vi "Main.vi"() -> ()   [LabVIEW 2021, in "Example Plugin.lvlib"]
doc: "This template is for the Queued Message Handler design pattern.\n\nThe Event Handling Loop generates messages based on user interface actions.\n\nThe Message Handling Loop processes messages generated by the Event Handling Loop, or by other messages. The messages are string values, so new messages can be added easily to the Message Cases case structure in the Message Handling Loop. Each message cluster can also provide an optional value for Message Data, which is a variant that can be converted to whatever message-specific data is required."
uses:
  Example Plugin.lvlib
  <vilib>/Plug-In SDKs/InstrumentStudio SDK/InstrumentStudioPluginSDK.lvlibp/Plugin Events Enum.ctl
  controls/Configuration.ctl
  377644f2-3ba0-40c2-9637-345728516e3e.vi
  dd0e9e37-20d8-45cf-b11e-f419cd56f172.vi
  377644f2-3ba0-40c2-9637-345728516e3e.vi/6651a77e-856e-4bcd-af5a-c0c13b264cc1.vi
  dd0e9e37-20d8-45cf-b11e-f419cd56f172.vi/331b549c-fcf8-43d9-8a1e-5b3c0091a99c.vi
  subVIs/Message Queue/Enqueue Message (Single).vi
  <vilib>/JDP Science/JSONtext/JSON text to Variant.vi
  <vilib>/Utility/error.llb/Error Cluster From Error Code.vi
  <vilib>/Plug-In SDKs/InstrumentStudio SDK/InstrumentStudioPluginSDK.lvlibp/Read Run Time Configuration.vi
  <vilib>/Plug-In SDKs/InstrumentStudio SDK/InstrumentStudioPluginSDK.lvlibp/Write Run Time Configuration.vi
  <vilib>/JDP Science/JSONtext/Variant to JSON Text.vi
  <vilib>/JDP Science/JSONtext/LVClass Serializer/JSONtext LVClass Serializer.lvclass
  <vilib>/ErrorRing/Error Ring.xnode
  <vilib>/Plug-In SDKs/InstrumentStudio SDK/InstrumentStudioPluginSDK.lvlibp/Plugin Session.lvclass
  <vilib>/Plug-In SDKs/InstrumentStudio SDK/InstrumentStudioPluginSDK.lvlibp
panel:
  in  "Tab Control 2":T1(tab)
  out "Project Path":path
  in  "Run Write":string
  in  "Write Run Time Config":bool
  in  "Edit Write":string
  in  "Write Edit Time Config":bool
  out "Run Read":string
  in  "Read Run Time Config":bool
  out "Edit Read":string
  in  "Read Edit Time Config":bool
  in  "Read Project Path":bool
  in  "Running":bool
  out "Event Record":i32(listbox)
  in  "Session Id":u64
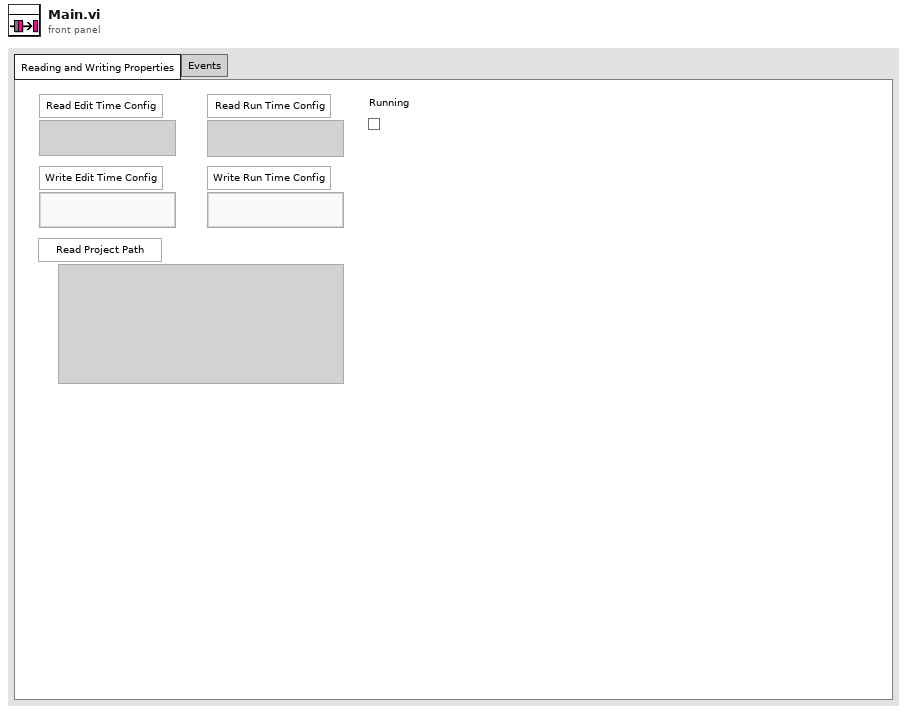
[diagram p1: front panel]
types:
  T1 = enum32{"Reading and Writing Properties", "Events"}
  T2 = typedef "Example Plugin.lvlib/Configuration.ctl" = cluster{"Edit Time Config":string, "Run Time Config":string, "Project Path":path}
  T3 = typedef "InstrumentStudioPluginSDK.lvlibp/Plugin Events Enum.ctl" = enum16{"Shutdown", "Project Saved", "Stop All Outputs"}
  T4 = typedef "InstrumentStudioPluginSDK.lvlibp/Event Registration Refnum.ctl" = refnum<event-registration>
  T5 = typedef "Example Plugin.lvlib/All Message Queues.ctl" = cluster{"UI":refnum<queue>}
  T6 = cluster{"Event Refnum":T4, "Event Registration Refnum":refnum<event-registration>}
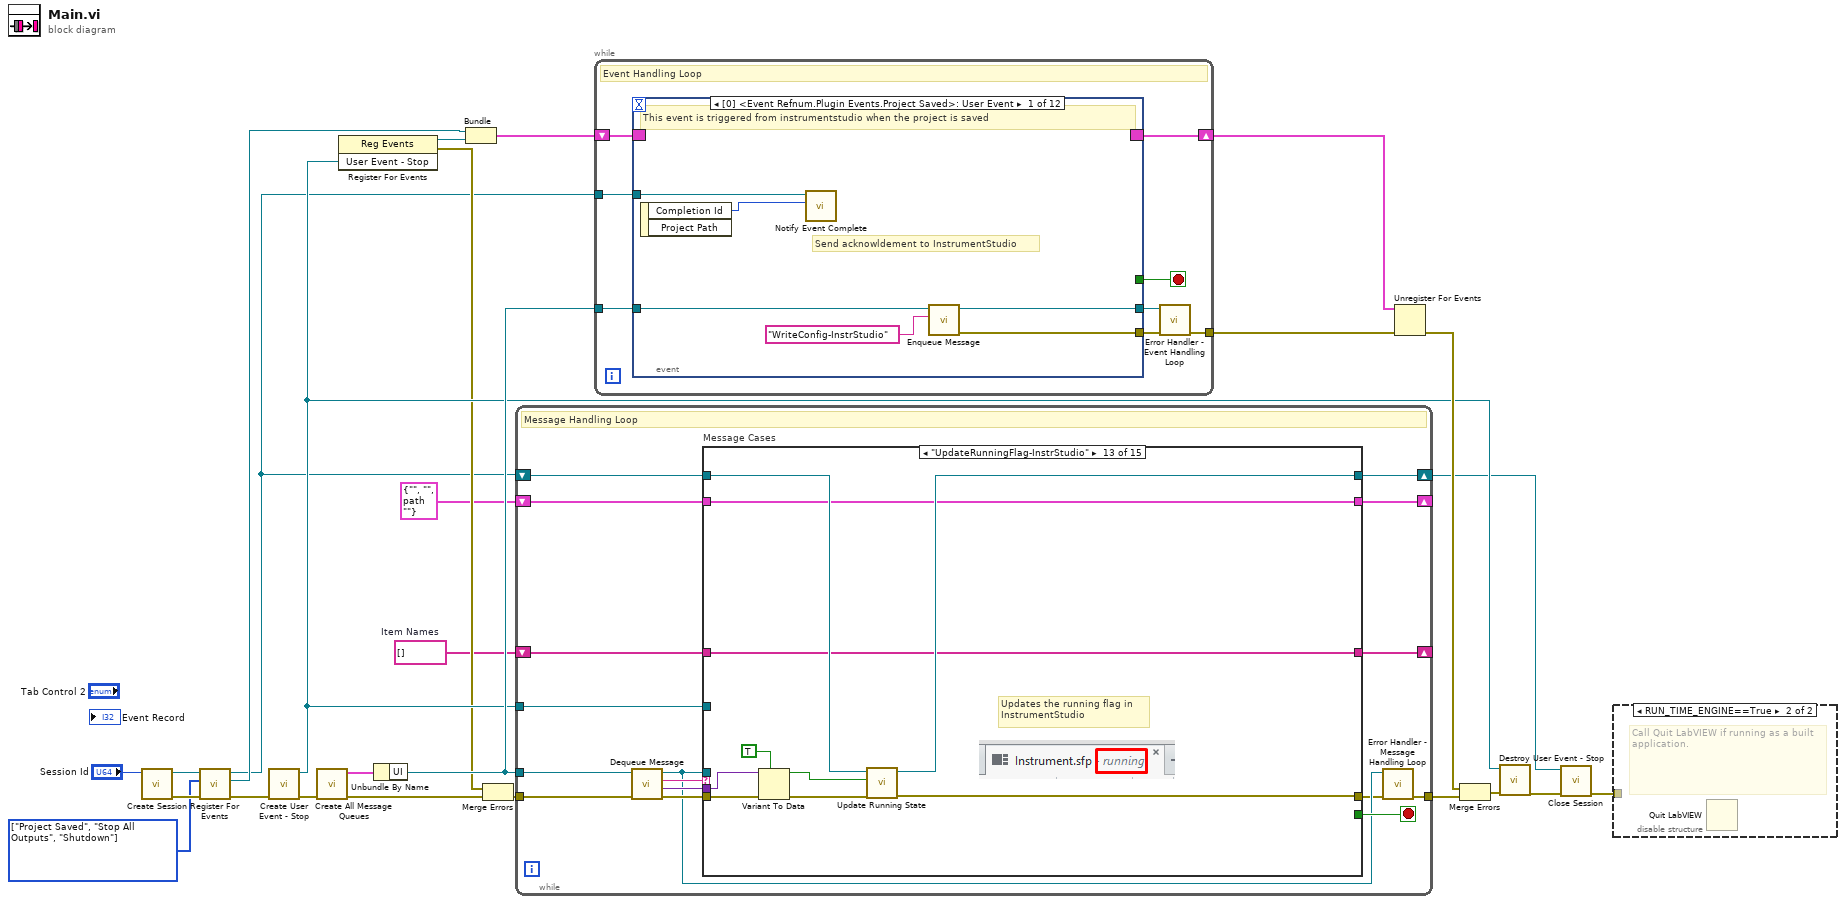
[diagram p0: block diagram]
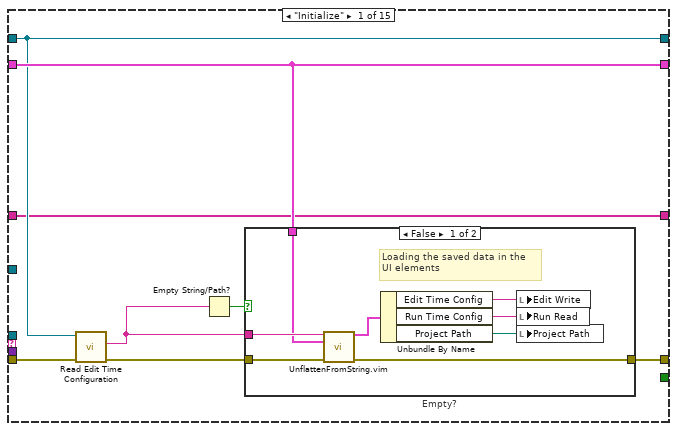
[diagram p3: hidden frame]
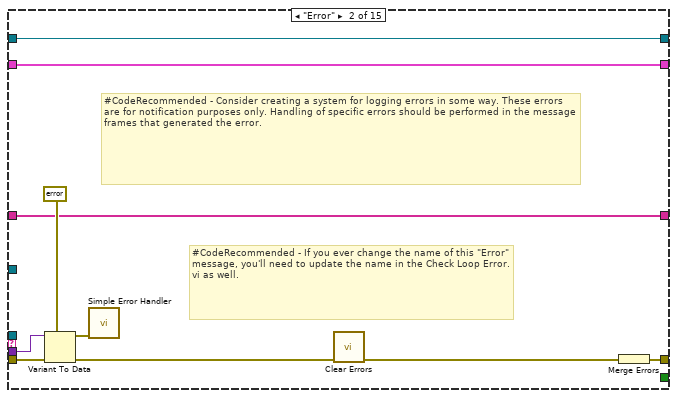
[diagram p5: hidden frame]
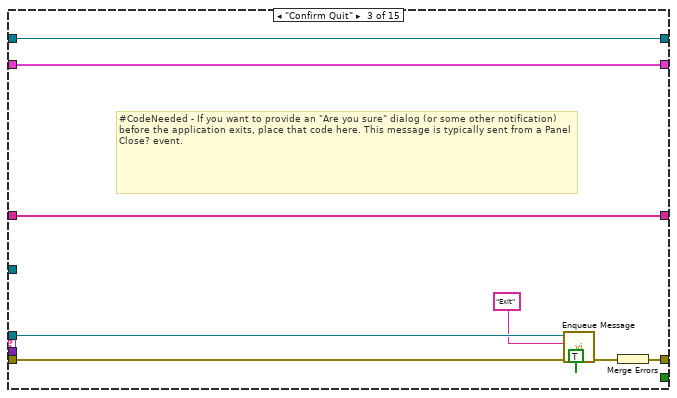
[diagram p6: hidden frame]
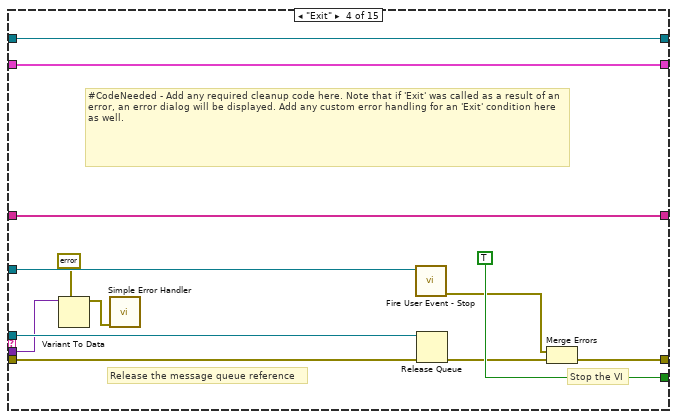
[diagram p7: hidden frame]
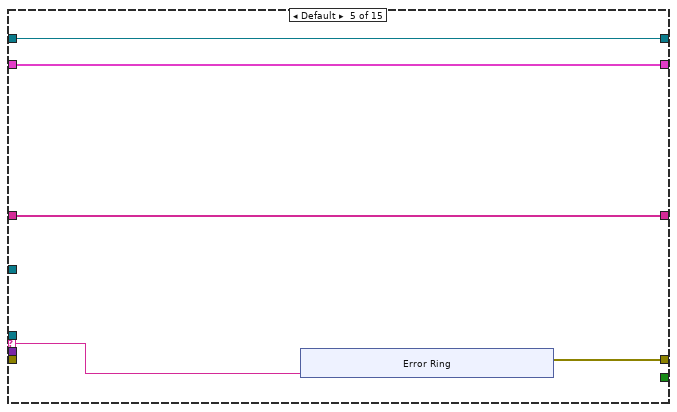
[diagram p8: hidden frame]
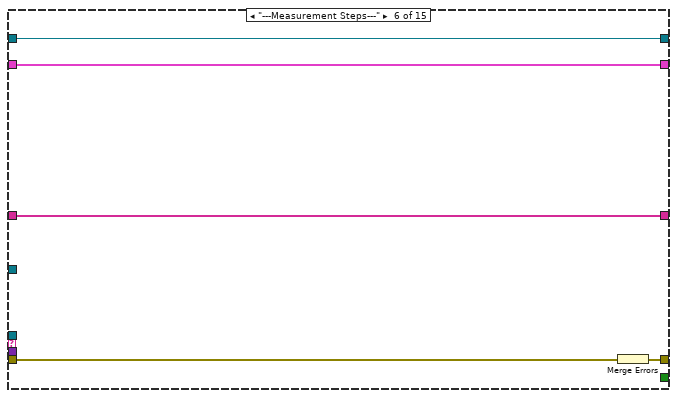
[diagram p9: hidden frame]
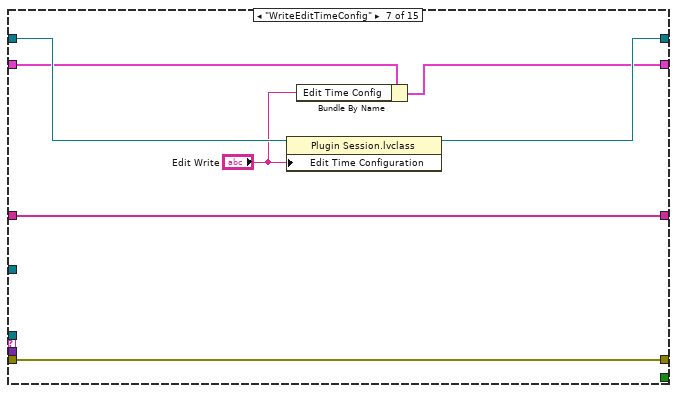
[diagram p10: hidden frame]
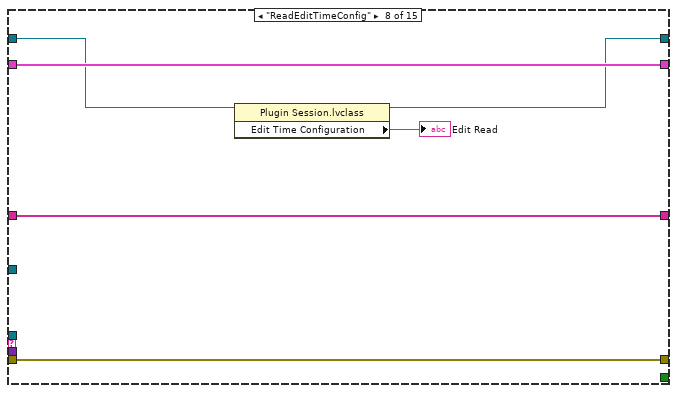
[diagram p11: hidden frame]
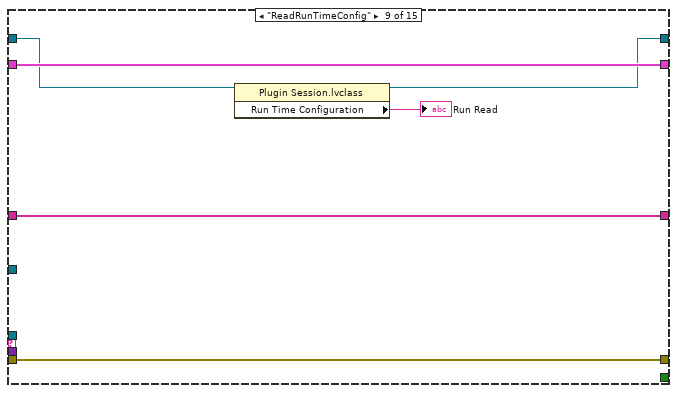
[diagram p12: hidden frame]
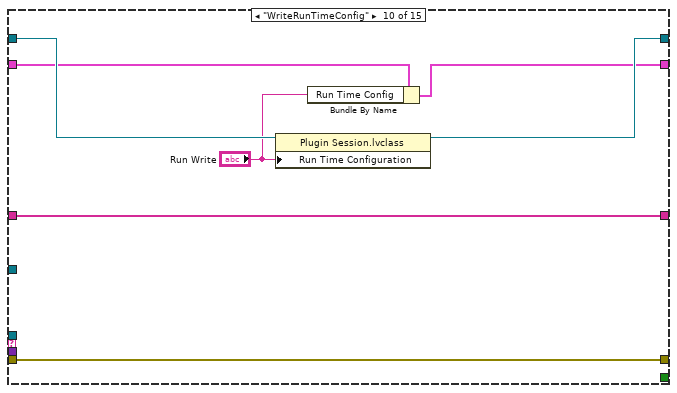
[diagram p13: hidden frame]
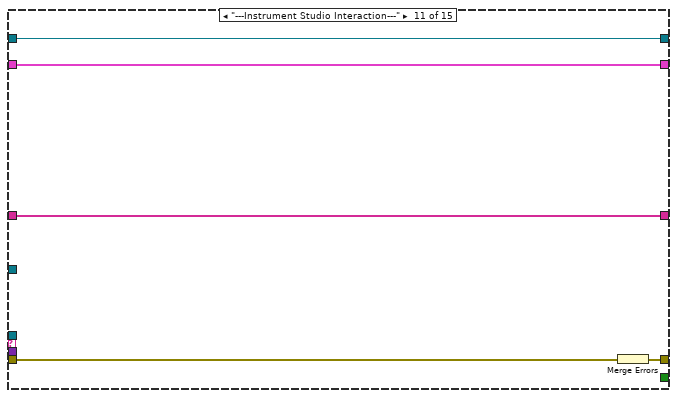
[diagram p14: hidden frame]
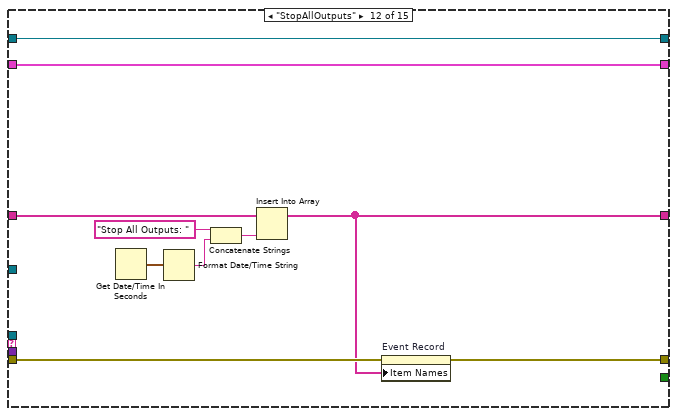
[diagram p15: hidden frame]
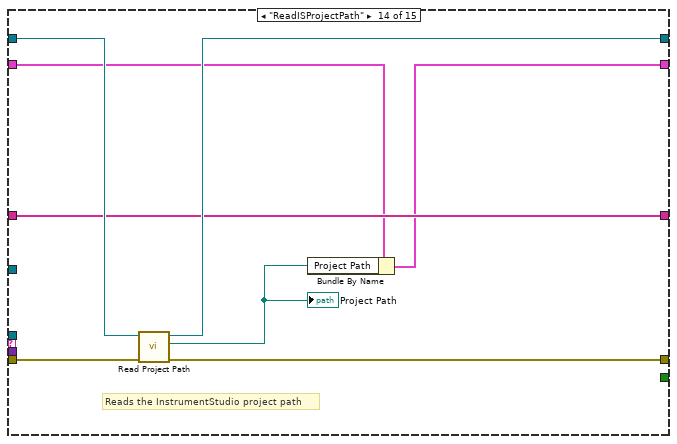
[diagram p16: hidden frame]
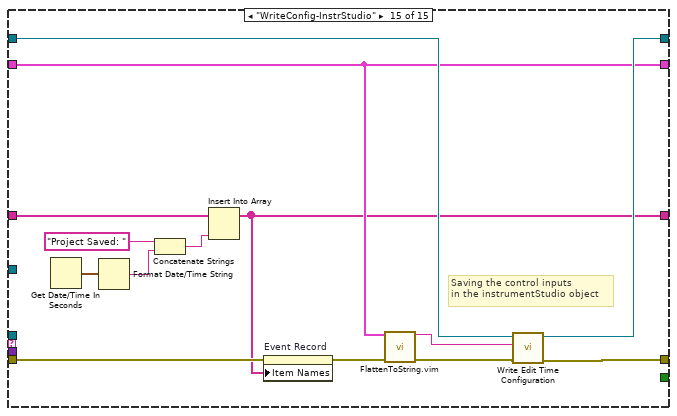
[diagram p17: hidden frame]
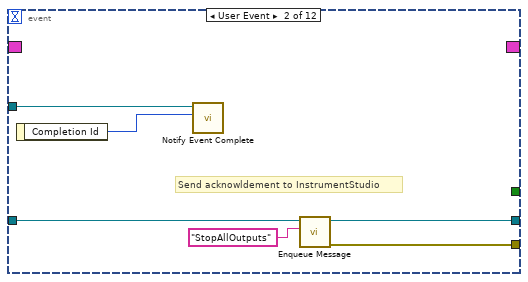
[diagram p18: hidden frame]
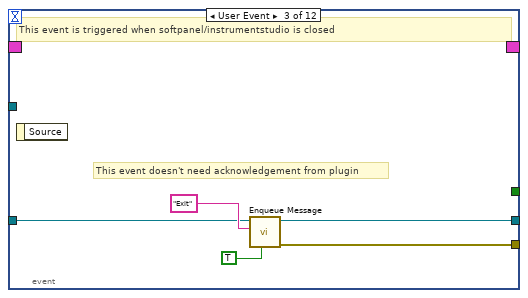
[diagram p19: hidden frame]
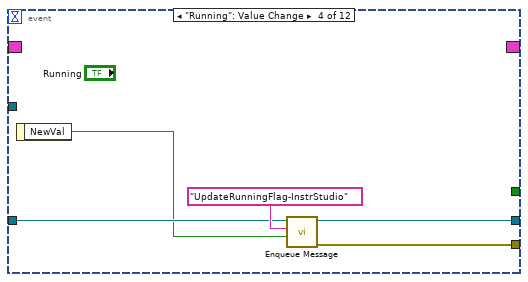
[diagram p20: hidden frame]
diagram:
  w1 = string[] []  # Item Names
  w10 = T3[] [enum."Project Saved", enum."Stop All Outputs", enum."Shutdown"] items=["Shutdown", "Project Saved", "Stop All Outputs"] ("Events To Register")
  n1 = call <vilib>:"Create Session.vi"("Session Id"="Session Id") -> ("error out"=w13:errorcluster, "Session out"=w11:refnum<class "Plugin Session.lvclass">)  [unwired: 6 in, 3 out]
  n2 = call <vilib>:"Register For Events.vi"("error in (no error)"=w13, "Events To Register"=w10, "Session in"=w11) -> ("error out"=w12:errorcluster, "Event Refnum"=w7:T4, "Session out"=w3:refnum<class "Plugin Session.lvclass">)  [unwired: 6 in]
  n3 = call "Create User Event - Stop.vi"("error in (no error)"=w12) -> ("error out"=w22:errorcluster, "User Event - Stop"=w17:refnum<user-event>)  [unwired: 9 in]
  n4 = call "Create All Message Queues.vi"("error in (no error)"=w22) -> ("error out"=w26:errorcluster, "Message Queues out"=w25:T5)  [unwired: 9 in]
  n5 = register-events(w17) -> (reference out=w9:refnum<event-registration>, error out=w15:errorcluster)  [unwired: 2 in]
  n6 = Unbundle By Name(w25) -> ("UI"=w23:refnum<queue>)
  n7 = Bundle("Event Refnum"=w7, "Event Registration Refnum"=w9) -> (w8:T6)  [unwired: 1 in]
  n8 = Merge Errors(w15, w26) -> (w16:errorcluster)
  n9 = while {
    tunnel: w23 -> [w36]
    tunnel: w17 -> [w41]
    tunnel: w16 -> [w40]
    tunnel: [w34] -> w24
    shift-right: [w31] -> w6
    shift-left: w3 -> [w32]
    shift-right: [w30] -> _
    shift-left: T2 {"Edit Time Config"="", "Run Time Config"="", "Project Path"=path ""} ("Configuration") -> [w29]
    shift-right: [w27] -> _
    shift-left: w1 -> [w28]
    stop <- w42 stop-if-true
    # "Message Handling Loop"
    n10 = call "Dequeue Message.vi"("error in (no error)"=w40, "Message Queue"=w36) -> ("error out"=w39:errorcluster, "Message Data"=w37:variant, "Message"=w38:string, "dup Message Queue"=w35:refnum<queue>)  [unwired: 6 in]
    n11 = case "Message Cases" shown="\"UpdateRunningFlag-InstrStudio\"" w38 {
      selector: w38 -> [_ _ _ _ w95 _ _ _ _ _ _ _ _ _ _]
      tunnel: w35 -> [_ _ w75 w91 _ _ _ _ _ _ _ _ _ _ _]
      tunnel: w39 -> [w44 w69 w78 w85 _ w108 w115 w121 w127 w134 w139 w141 w156 w166 w170]
      tunnel: [w49 w64 w77 w88 w96 w107 w115 w121 w127 w134 w138 w142 w157 w164 w179] -> w33
      tunnel: [_ _ _ TRUE _ _ _ _ _ _ _ _ _ _ _] -> w42
      tunnel: w37 -> [_ w68 _ w82 _ _ _ _ _ _ _ _ w155 _ _]
      tunnel: w41 -> [_ _ _ w87 _ _ _ _ _ _ _ _ _ _ _]
      tunnel: w32 -> [w47 w63 w72 w81 w94 w106 w113 w118 w124 w132 w137 w149 w159 w167 w181]
      tunnel: [w47 w63 w72 w81 w94 w106 w114 w119 w125 w133 w137 w149 w158 w165 w180] -> w31
      tunnel: [w50 w62 w71 w80 w93 w105 w112 w120 w126 w130 w136 w148 w151 w161 w176] -> w30
      tunnel: w29 -> [w50 w62 w71 w80 w93 w105 w111 w120 w126 w129 w136 w148 w151 w160 w176]
      tunnel: w28 -> [w43 w60 w70 w79 w92 w104 w109 w116 w122 w128 w135 w143 w150 w163 w169]
      tunnel: [w43 w60 w70 w79 w92 w104 w109 w116 w122 w128 w135 w140 w150 w163 w168] -> w27
      frame "Initialize" {
        # "Initialize - All initialization work should take place in this message, since other loops can potentially enqueue messages that execute immediately after this one."
        n12 = call <vilib>:"Read Edit Time Configuration.vi"("error in (no error)"=w44, "Session in"=w47) -> ("error out"=w45:errorcluster, "Edit Time Configuration"=w46:string)  [unwired: 7 in, 1 out]
        n13 = Empty String/Path?(string/path=w46) -> (empty?=w48:bool)
        n14 = case "Empty?" shown="False" w48 {
          tunnel: w50 -> [w57 _]
          tunnel: [w55 w59] -> w49
          tunnel: w45 -> [w54 w59]
          tunnel: w46 -> [w58 _]
          frame False {
            # "Loading the saved data in the \nUI elements"
            n15 = call "UnflattenFromString.vim"("Flattened Data"=w58, "Data Type"=w57, "error in"=w54) -> ("Data Out"=w56:T2, "error out"=w55:errorcluster)  [unwired: 11 in]
            n16 = Unbundle By Name(w56) -> ("Edit Time Config"=w53:string, "Run Time Config"=w52:string, "Project Path"=w51:path)
            n17 = local write "Edit Write"(w53) -> ()
            n18 = local write "Run Read"(w52) -> ()
            n19 = local write "Project Path"(w51) -> ()
          }
          frame True {
          }
        }
      }
      frame "Error" {
        # "#CodeRecommended - If you ever change the name of this \"Error\" message, you'll need to update the name in the Check Loop Error.vi as well."
        # "#CodeRecommended - Consider creating a system for logging errors in some way. These errors are for notification purposes only. Handling of specific errors should be performed in the message frames that generated the error."
        # "Error - Display an error dialog. This message is sent by the \"Error Handler\" VIs at the end of other loops in this application."
        n20 = Variant To Data(error in=w69, type=errorcluster {"status"=FALSE, "code"=0, "source"=""} ("error constant"), Variant=w68) -> (data=w66:errorcluster, error out=w65:errorcluster)
        n21 = call <vilib>:"Simple Error Handler.vi"("error in (no error)"=w66) -> ()  [unwired: 4 in, 5 out]
        n22 = call <vilib>:"Clear Errors.vi"("error in (no error)"=w65) -> ("error out"=w61:errorcluster)  [unwired: 5 in, 1 out]
        n23 = Merge Errors(w61) -> (w64:errorcluster)
      }
      frame "Confirm Quit" {
        # "#CodeNeeded - If you want to provide an \"Are you sure\" dialog (or some other notification) before the application exits, place that code here. This message is typically sent from a Panel Close? event."
        # "Confirm Quit - Message that can confirm whether or not the user wants to exit the application."
        n24 = call-poly "Enqueue Message.vi"("Priority Message? (F)"=TRUE, "error in (no error)"=w78, "Message"="Exit", "Message Queue"=w75) -> ("error out"=w76:errorcluster)  [unwired: 6 in, 1 out]
        n25 = Merge Errors(w76) -> (w77:errorcluster)
      }
      frame "Exit" {
        # "Stop the VI"
        # "Release the message queue reference"
        # "#CodeNeeded - Add any required cleanup code here. Note that if 'Exit' was called as a result of an error, an error dialog will be displayed. Add any custom error handling for an 'Exit' condition here as well."
        # "Exit - Exit the application."
        n26 = Variant To Data(type=errorcluster {"status"=FALSE, "code"=0, "source"=""} ("error constant"), Variant=w82) -> (data=w83:errorcluster)  [unwired: 1 in, 1 out]
        n27 = call <vilib>:"Simple Error Handler.vi"("error in (no error)"=w83) -> ()  [unwired: 4 in, 5 out]
        n28 = call "Fire User Event - Stop.vi"("User Event - Stop"=w87) -> ("error out"=w86:errorcluster)  [unwired: 10 in]
        n29 = Release Queue(queue=w91, error in (no error)=w85) -> (error out=w89:errorcluster)  [unwired: 1 in, 2 out]
        n30 = Merge Errors(w86, w89) -> (w88:errorcluster)
      }
      frame Default {
        # "'Default' case only runs if there is a message that isn't defined in any of the other cases.  Output a programming error."
        n31 = xnode "Error Ring"("parameter 0"=w95) -> ("error out"=w96:errorcluster)
      }
      frame "---Measurement Steps---" {
        # "Duplicate this frame when creating new messages.  Change this comment in the duplicated frame to describe this message."
        n32 = Merge Errors(w108) -> (w107:errorcluster)
      }
      frame "WriteEditTimeConfig" {
        n33 = property class="Plugin Session.lvclass"(reference=w113, "Edit Time Configuration"="Edit Write") -> (reference out=w114:refnum<class "Plugin Session.lvclass">)  [unwired: 1 in, 1 out]
        n34 = Bundle By Name(cluster=w111, "Edit Time Config"="Edit Write") -> (w112:T2)
      }
      frame "ReadEditTimeConfig" {
        n35 = property class="Plugin Session.lvclass"(reference=w118) -> (reference out=w119:refnum<class "Plugin Session.lvclass">, "Edit Time Configuration"=→"Edit Read":string)  [unwired: 1 in, 1 out]
      }
      frame "ReadRunTimeConfig" {
        n36 = property class="Plugin Session.lvclass"(reference=w124) -> (reference out=w125:refnum<class "Plugin Session.lvclass">, "Run Time Configuration"=→"Run Read":string)  [unwired: 1 in, 1 out]
      }
      frame "WriteRunTimeConfig" {
        n37 = property class="Plugin Session.lvclass"(reference=w132, "Run Time Configuration"="Run Write") -> (reference out=w133:refnum<class "Plugin Session.lvclass">)  [unwired: 1 in, 1 out]
        n38 = Bundle By Name(cluster=w129, "Run Time Config"="Run Write") -> (w130:T2)
      }
      frame "---Instrument Studio Interaction---" {
        # "Duplicate this frame when creating new messages.  Change this comment in the duplicated frame to describe this message."
        n39 = Merge Errors(w139) -> (w138:errorcluster)
      }
      frame "StopAllOutputs" {
        n40 = Get Date/Time In Seconds() -> (seconds since 1Jan1904=w144:timestamp)
        n41 = Format Date/Time String(seconds (now)=w144) -> (date/time string=w146:string)  [unwired: 2 in]
        n42 = Concatenate Strings("Stop All Outputs: ", w146) -> (w145:string)
        n43 = Insert Into Array(array=w143, new element=w145) -> (w140:string[])  [unwired: 1 in]
        n44 = property on="Event Record" class="LstBox (strict)"(error in=w141, "Item Names"=w140) -> (error out=w142:errorcluster)  [unwired: 1 in, 1 out]
      }
      frame "UpdateRunningFlag-InstrStudio" {
        # "Updates the running flag in \nInstrumentStudio"
        n45 = Variant To Data(error in=w156, type=TRUE, Variant=w155) -> (data=w153:bool, error out=w152:errorcluster)
        n46 = call <vilib>:"Update Running State.vi"("error in (no error)"=w152, "Is Running"=w153, "Plugin Session in"=w159) -> ("error out"=w157:errorcluster, "Plugin Session out"=w158:refnum<class "Plugin Session.lvclass">)  [unwired: 7 in]
      }
      frame "ReadISProjectPath" {
        # "Reads the InstrumentStudio project path"
        n47 = call <vilib>:"Read Project Path.vi"("error in (no error)"=w166, "Session in"=w167) -> ("error out"=w164:errorcluster, "Project Path"=w162:path, "Session out"=w165:refnum<class "Plugin Session.lvclass">)  [unwired: 7 in]
        "Project Path" <- w162
        n48 = Bundle By Name(cluster=w160, "Project Path"=w162) -> (w161:T2)
      }
      frame "WriteConfig-InstrStudio" {
        # "Saving the control inputs\nin the instrumentStudio object"
        n49 = Get Date/Time In Seconds() -> (seconds since 1Jan1904=w173:timestamp)
        n50 = Format Date/Time String(seconds (now)=w173) -> (date/time string=w175:string)  [unwired: 2 in]
        n51 = Concatenate Strings("Project Saved: ", w175) -> (w174:string)
        n52 = Insert Into Array(array=w169, new element=w174) -> (w168:string[])  [unwired: 1 in]
        n53 = property on="Event Record" class="LstBox (strict)"(error in=w170, "Item Names"=w168) -> (error out=w171:errorcluster)  [unwired: 1 in, 1 out]
        n54 = call "FlattenToString.vim"("Anything"=w176, "error in"=w171) -> ("Flattened Data"=w178:string, "error out"=w177:errorcluster)  [unwired: 12 in]
        n55 = call <vilib>:"Write Edit Time Configuration.vi"("error in (no error)"=w177, "Edit Time Configuration"=w178, "Session in"=w181) -> ("error out"=w179:errorcluster, "Session out"=w180:refnum<class "Plugin Session.lvclass">)  [unwired: 7 in]
      }
    }
    n56 = call "Error Handler - Message Handling Loop.vi"("error in (no error)"=w33, "Message Queue"=w35) -> ("dup error in"=w34:errorcluster)  [unwired: 8 in, 1 out]
  }
  n57 = while {
    tunnel: w23 -> [w189]
    shift-right: [w187] -> w19
    shift-left: w8 -> [w188]
    tunnel: [w183] -> w18
    tunnel: w3 -> [w182]
    stop <- w185 stop-if-true
    # "Event Handling Loop"
    n58 = event shown="[0] <Event Refnum.Plugin Events.Project Saved>: User Event" {
      selector: w188 -> [_ _ _ _ _ _ _ _ _ _ _ _]
      dyn-events: [_ _ _ _ _ _ _ _ _ _ _ _] -> w187
      timeout: _ -> [_ _ _ _ _ _ _ _ _ _ _ _]
      tunnel: [_ _ _ _ _ _ _ _ _ _ _ TRUE ("Discard?")] -> w185
      tunnel: w189 -> [w192 w199 w202 w210 w214 w218 w220 w223 w225 w232 w234 w236]
      tunnel: [w190 w196 w203 w208 w213 _ _ _ _ w231 _ _] -> w186
      tunnel: [w191 w197 w204 w209 w215 w217 w219 w222 w226 w230 w234 w236] -> w184
      tunnel: w182 -> [w195 w201 _ _ _ _ _ _ _ _ _ _]
      event User Event {
        # "Send acknowldement to InstrumentStudio"
        # "This event is triggered from instrumentstudio when the project is saved"
        n59 = event-data() -> ("Completion Id"=w194:i64)  [unwired: 1 in, 1 out]
        n60 = call <vilib>:"Notify Event Complete.vi"("Completion Id"=w194, "Session in"=w195) -> ()  [unwired: 8 in, 2 out]
        n61 = call-poly "Enqueue Message.vi"("Message"="WriteConfig-InstrStudio", "Message Queue"=w192) -> ("error out"=w190:errorcluster, "dup Message Queue"=w191:refnum<queue>)  [unwired: 8 in]
      }
      event User Event {
        # "Send acknowldement to InstrumentStudio"
        n62 = event-data() -> ("Completion Id"=w200:i64)  [unwired: 1 in]
        n63 = call <vilib>:"Notify Event Complete.vi"("Completion Id"=w200, "Session in"=w201) -> ()  [unwired: 8 in, 2 out]
        n64 = call-poly "Enqueue Message.vi"("Message"="StopAllOutputs", "Message Queue"=w199) -> ("error out"=w196:errorcluster, "dup Message Queue"=w197:refnum<queue>)  [unwired: 8 in]
      }
      event User Event {
        # "This event doesn't need acknowledgement from plugin"
        # "This event is triggered when softpanel/instrumentstudio is closed"
        n65 = event-data() -> ()  [unwired: 1 in, 1 out]
        n66 = call-poly "Enqueue Message.vi"("Priority Message? (F)"=TRUE, "Message"="Exit", "Message Queue"=w202) -> ("error out"=w203:errorcluster, "dup Message Queue"=w204:refnum<queue>)  [unwired: 7 in]
      }
      event "Running": Value Change {
        n67 = event-data() -> ("NewVal"=w207:bool)  [unwired: 1 in]
        n68 = call-poly "Enqueue Message.vi"("Message Data"=w207, "Message"="UpdateRunningFlag-InstrStudio", "Message Queue"=w210) -> ("error out"=w208:errorcluster, "dup Message Queue"=w209:refnum<queue>)  [unwired: 7 in]
      }
      event "Read Project Path": Value Change {
        n69 = event-data() -> ()  [unwired: 1 in, 1 out]
        n70 = call-poly "Enqueue Message.vi"("Message"="ReadISProjectPath", "Message Queue"=w214) -> ("error out"=w213:errorcluster, "dup Message Queue"=w215:refnum<queue>)  [unwired: 8 in]
      }
      event "Write Edit Time Config": Value Change {
        n71 = event-data() -> ()  [unwired: 1 in, 1 out]
        n72 = call-poly "Enqueue Message.vi"("Message"="WriteEditTimeConfig", "Message Queue"=w218) -> ("dup Message Queue"=w217:refnum<queue>)  [unwired: 8 in, 1 out]
      }
      event "Read Edit Time Config": Value Change {
        n73 = event-data() -> ()  [unwired: 1 in, 1 out]
        n74 = call-poly "Enqueue Message.vi"("Message"="ReadEditTimeConfig", "Message Queue"=w220) -> ("dup Message Queue"=w219:refnum<queue>)  [unwired: 8 in, 1 out]
      }
      event "Read Run Time Config": Value Change {
        n75 = event-data() -> ()  [unwired: 1 in, 1 out]
        n76 = call-poly "Enqueue Message.vi"("Message"="ReadRunTimeConfig", "Message Queue"=w223) -> ("dup Message Queue"=w222:refnum<queue>)  [unwired: 8 in, 1 out]
      }
      event "Write Run Time Config": Value Change {
        n77 = event-data() -> ()  [unwired: 1 in, 1 out]
        n78 = call-poly "Enqueue Message.vi"("Message"="WriteRunTimeConfig", "Message Queue"=w225) -> ("dup Message Queue"=w226:refnum<queue>)  [unwired: 8 in, 1 out]
      }
      event Panel Close? {
        # "Send the 'Confirm Quit' message if the user closes the panel of the VI. Discard the event so the 'Confirm Quit' message has a chance to run."
        n79 = event-data() -> ()  [unwired: 1 in, 1 out]
        n80 = call-poly "Enqueue Message.vi"("Priority Message? (F)"=TRUE, "Message"="Confirm Quit", "Message Queue"=w232) -> ("error out"=w231:errorcluster, "dup Message Queue"=w230:refnum<queue>)  [unwired: 7 in]
        n81 = event-data("Discard?"=TRUE) -> ()  [unwired: 1 in, 1 out]
      }
      event Application Instance Close {
        # "#CodeRecommended - When a project closes, all VIs within that project are aborted and leave memory. However, any code placed in this event frame is guaranteed to run to completion, so add any cleanup code that absolutely must happen here."
        n82 = event-data() -> ()  [unwired: 1 in, 1 out]
      }
      event User Event {
        # "The Message Handling Loop processed an \"Exit\" message, which fired this event to stop the Event Handling Loop."
        n83 = event-data() -> ()  [unwired: 1 in, 1 out]
      }
    }
    n84 = call "Error Handler - Event Handling Loop.vi"("error in (no error)"=w186, "Message Queue"=w184) -> ("dup error in"=w183:errorcluster)  [unwired: 8 in, 1 out]
  }
  n85 = Unregister For Events(event registration refnum=w19, error in=w18) -> (error out=w20:errorcluster)
  n86 = Merge Errors(w20, w24) -> (w21:errorcluster)
  n87 = call "Destroy User Event - Stop.vi"("error in (no error)"=w21, "User Event - Stop"=w17) -> ("error out"=w5:errorcluster)  [unwired: 9 in]
  n88 = call <vilib>:"Close Session.vi"("error in (no error)"=w5, "Session in"=w6) -> ("error out"=w4:errorcluster)  [unwired: 9 in]
  n89 = disable-structure shown="RUN_TIME_ENGINE==True" {
    disable-tunnel: w4 -> [_ _]
    frame condition #0 (active) {
    }
    frame condition #1 {
      # "Call Quit LabVIEW if running as a built application."
      n90 = Quit LabVIEW() -> ()  [unwired: 1 in]
    }
  }
